vi "population_generation.vi"(0 "Zero Level on":bool, 1 "Array 3":dbl[](array[numeric]), 2 "Zero Ensemble Power":dbl, 3 "Saturation Polarization":dbl, 4 "Array 4":dbl[](array[numeric]), 5 "Array 2":dbl[](array[numeric]), 6 "Zero Ensemble Area":dbl, 8 "Array":dbl[](array[numeric]), 9 "Normed Array":dbl[](array[numeric]), 10 "Microwave Power":dbl, 11 "Normed Array 3":dbl[](array[numeric]), 12 "Microwave on":bool, 13 "Normed Array 2":dbl[](array[numeric]), 14 "Relaxation Rate":dbl) -> (18 "Zero Ensemble Out":dbl[](array[numeric]), 20 "rho- array out 2":dbl[](array[numeric]), 21 "rho+ array out":dbl[](array[numeric]), 22 "rho0 array out 2":dbl[](array[numeric]), 23 "rho- array out":dbl[](array[numeric]), 24 "rho+ array out 2":dbl[](array[numeric]), 25 "rho0 array out":dbl[](array[numeric]), 26 "rho0 decay out":dbl[](array[numeric]))   [LabVIEW 2018]
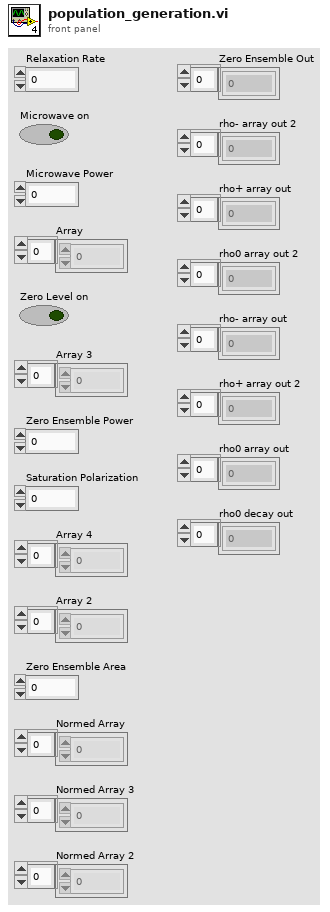
[diagram p1: front panel]
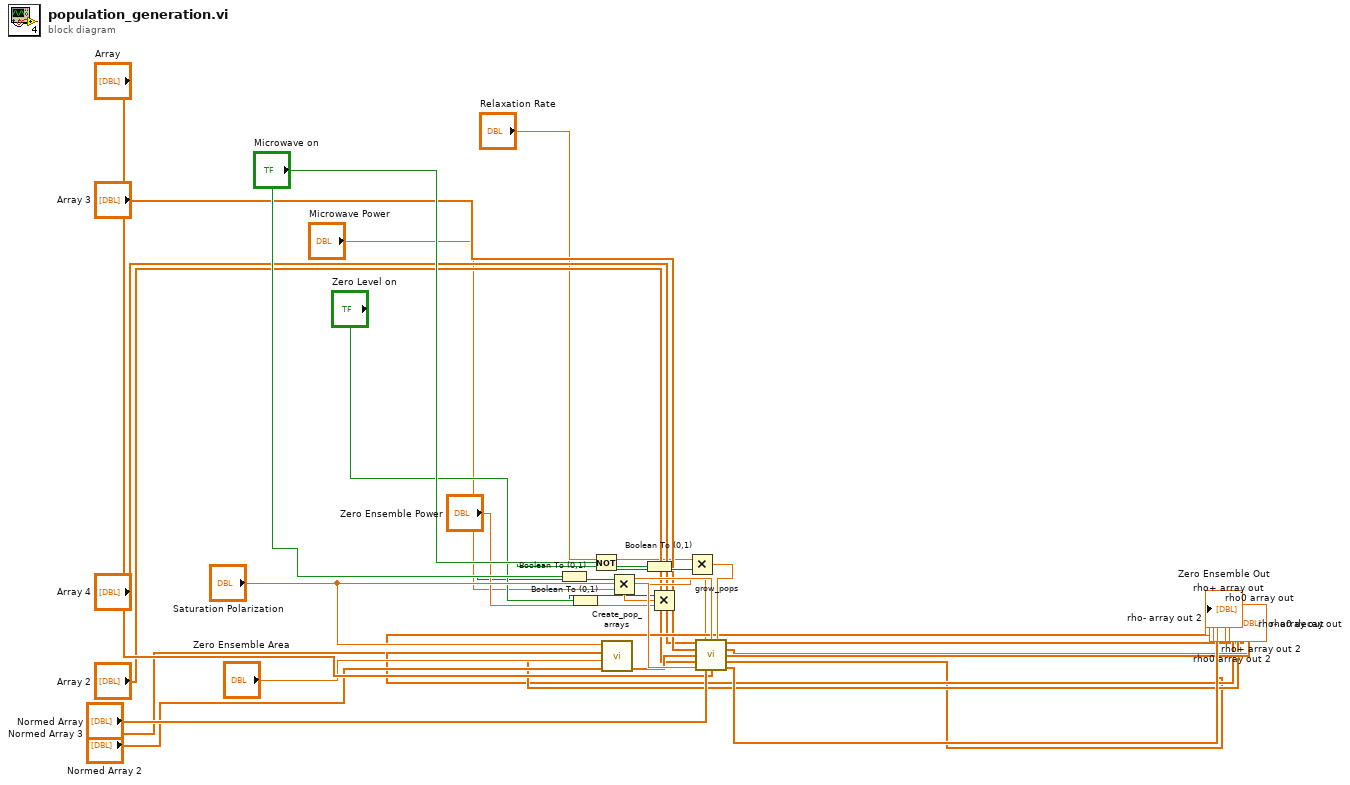
[diagram p0: block diagram]
diagram:
  n1 = Boolean To (0,1)(Boolean="Microwave on") -> (0, 1=w8:i16)
  n2 = Boolean To (0,1)(Boolean="Zero Level on") -> (0, 1=w17:i16)
  n3 = Not(x="Microwave on") -> (.not. x?=w29:bool)
  n4 = call "Create_pop_arrays.vi"("Zero ensemble in"="Normed Array 2", "Zero ensemble area in"="Zero Ensemble Area", "Normalized I in"="Normed Array 3", "Saturation Polarization"="Saturation Polarization") -> ("Zero ensemble out"=w16:dbl[], "rho- array out"=→"rho- array out":dbl[], "rho0 array out"=→"rho0 array out 2":dbl[], "rho+ array out"=→"rho+ array out":dbl[])  [unwired: 4 in]
  n5 = Multiply(x=w8, y="Microwave Power") -> (x*y=w7:dbl)
  n6 = Boolean To (0,1)(Boolean=w29) -> (0, 1=w28:i16)
  n7 = Multiply(x=w17, y="Zero Ensemble Power") -> (x*y=w18:dbl)
  n8 = Multiply(x="Relaxation Rate", y=w28) -> (x*y=w27:dbl)
  n9 = call "grow_pops.vi"("rho+ array"="Array 4", "Microwave power"=w7, "Zero Level Power"=w18, "Decay rate"=w27, "rho0 array"="Array 3", "Zero Ensemble Condition"=w16, "rho- array"="Array 2", "Sat pol"="Saturation Polarization", "I array"="Normed Array", "Zero Ensemble Array"="Array") -> ("rho+ array out"=→"rho+ array out 2":dbl[], "rho0 array out"=→"rho0 array out":dbl[], "rho0 decay out"=→"rho0 decay out":dbl[], "rho- array out"=→"rho- array out 2":dbl[], "Zero Ensemble Out"=→"Zero Ensemble Out":dbl[])  [unwired: 1 in]
